vi "SaveSpec.vi"(3 "其它规格":T6={"其它勾选类规格"={"保存图片"=FALSE, "上传设备状态数据"=FALSE, "保存数据"=FALSE, "开机默认开启监控摄像头"=FALSE, "启用mark拍照 "=FALSE}, "其它数据类规格"={"相机1像素-毫米换算系数"=15.0, "相机2像素-毫米换算系数"=15.0, "D盘剩余空间预警(G)"=15.0, "视频最长录制时间(秒)"=15.0}, "相机名称"={"相机1名称"="cam1", "相机2名称"="cam1", "Cam1启用"=FALSE, "Cam2启用"=FALSE, "Basler1"=FALSE, "Basler2"=FALSE}, "参数"={"Mark1曝光时间"=500, "Mark2曝光时间"=500, "二维码曝光时间"=500}} {"其它数据类规格"."视频最长录制时间(秒)" format="%.3f"; "其它数据类规格"."D盘剩余空间预警(G)" format="%.3f"; "其它数据类规格"."相机1像素-毫米换算系数" format="%.5f"; "其它数据类规格"."相机2像素-毫米换算系数" format="%.5f"}) -> (0 "File out":path)   [LabVIEW 2014]
uses:
  Controls/OtherSpec.ctl
  <vilib>/userdefined/High Color/IMAQdx.ctl
  Global.vi
  <vilib>/Utility/file.llb/Write To Spreadsheet File (string).vi
panel:
  out "输出数组":string[][](array[string])
  in  "参数":T1={"Mark1曝光时间"=500.0, "Mark2曝光时间"=500.0, "二维码曝光时间"=500.0}
  in  "相机名称":T2={"相机1名称"="cam1", "相机2名称"="cam1", "Cam1启用"=FALSE, "Cam2启用"=FALSE, "Basler1"=FALSE, "Basler2"=FALSE}
  in  "其它数据类规格":T4={"相机1像素-毫米换算系数"=15.0, "相机2像素-毫米换算系数"=15.0, "D盘剩余空间预警(G)"=15.0, "视频最长录制时间(秒)"=15.0} {"视频最长录制时间(秒)" format="%.3f"; "D盘剩余空间预警(G)" format="%.3f"; "相机1像素-毫米换算系数" format="%.5f"; "相机2像素-毫米换算系数" format="%.5f"}
  in  "其它勾选类规格":T5
  out "输出字符串 3":string
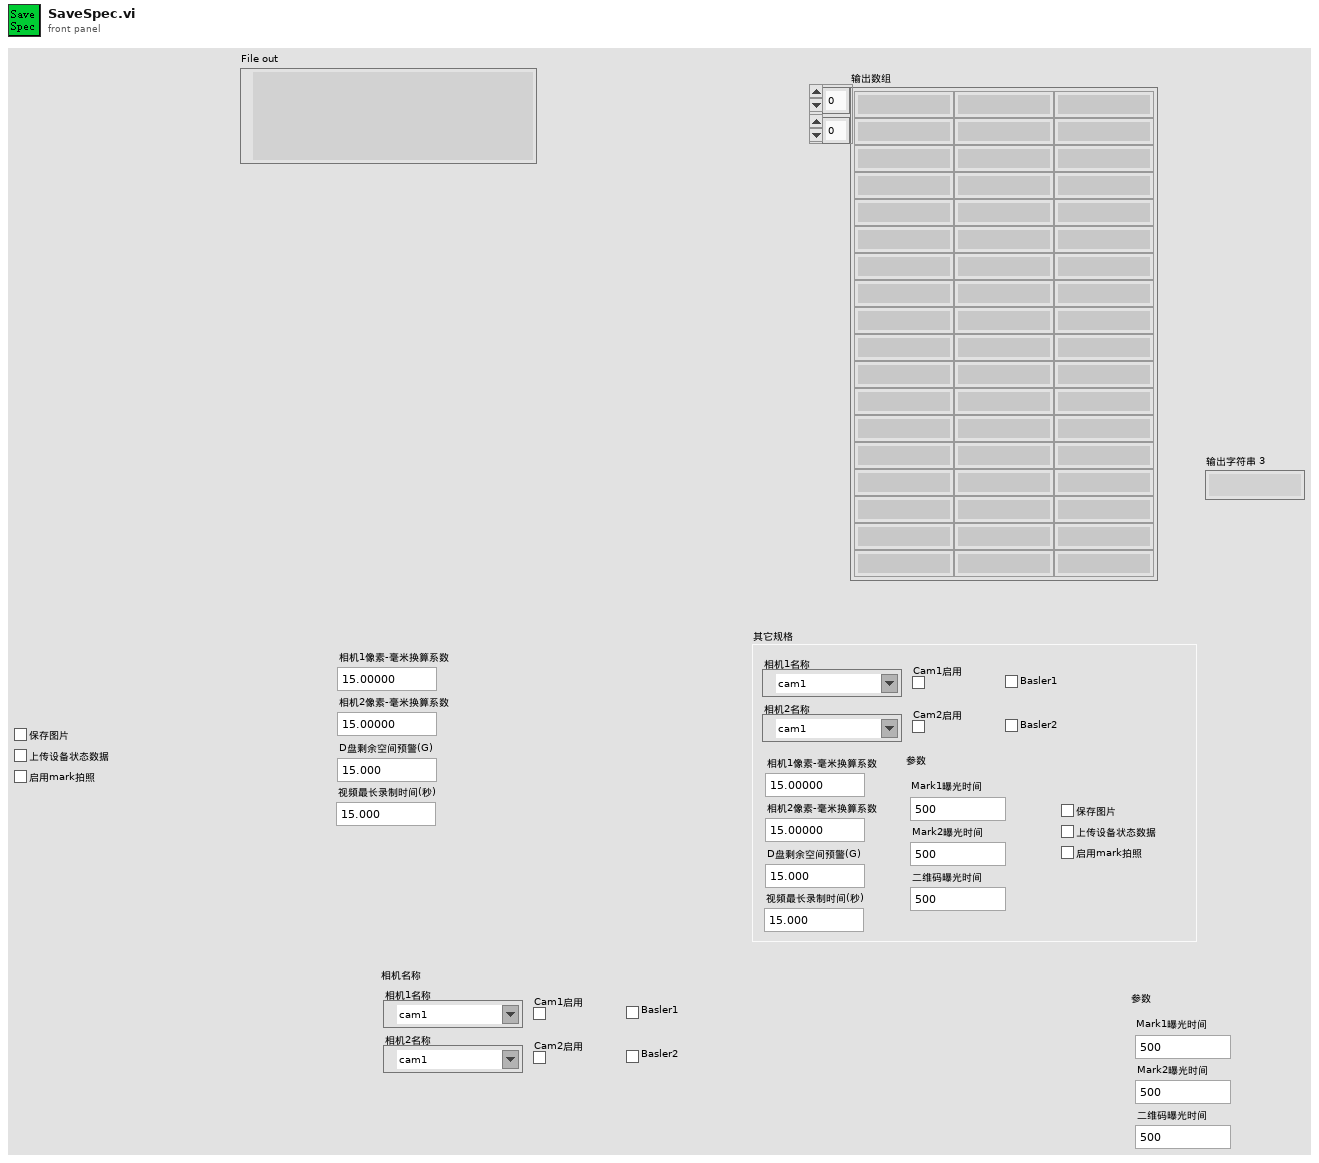
[diagram p1: front panel]
types:
  T1 = cluster{"Mark1曝光时间":dbl, "Mark2曝光时间":dbl, "二维码曝光时间":dbl}
  T2 = typedef "相机名称品牌使用状态.ctl" = cluster{"相机1名称":T3, "相机2名称":T3, "Cam1启用":bool, "Cam2启用":bool, "Basler1":bool, "Basler2":bool}
  T3 = typedef "IMAQdx.ctl" = refnum<k21>
  T4 = typedef "其他数据类规格.ctl" = cluster{"相机1像素-毫米换算系数":dbl, "相机2像素-毫米换算系数":dbl, "D盘剩余空间预警(G)":dbl, "视频最长录制时间(秒)":dbl}
  T5 = typedef "其它勾选类规格.ctl" = cluster{"保存图片":bool, "上传设备状态数据":bool, "保存数据":bool, "开机默认开启监控摄像头":bool, "启用mark拍照 ":bool}
  T6 = typedef "OtherSpec.ctl" = cluster{"其它勾选类规格":T5, "其它数据类规格":T4, "相机名称":T2, "参数":cluster{"Mark1曝光时间":i32, "Mark2曝光时间":i32, "二维码曝光时间":i32}}
  T7 = cluster{"Mark1曝光时间":i32, "Mark2曝光时间":i32, "二维码曝光时间":i32}
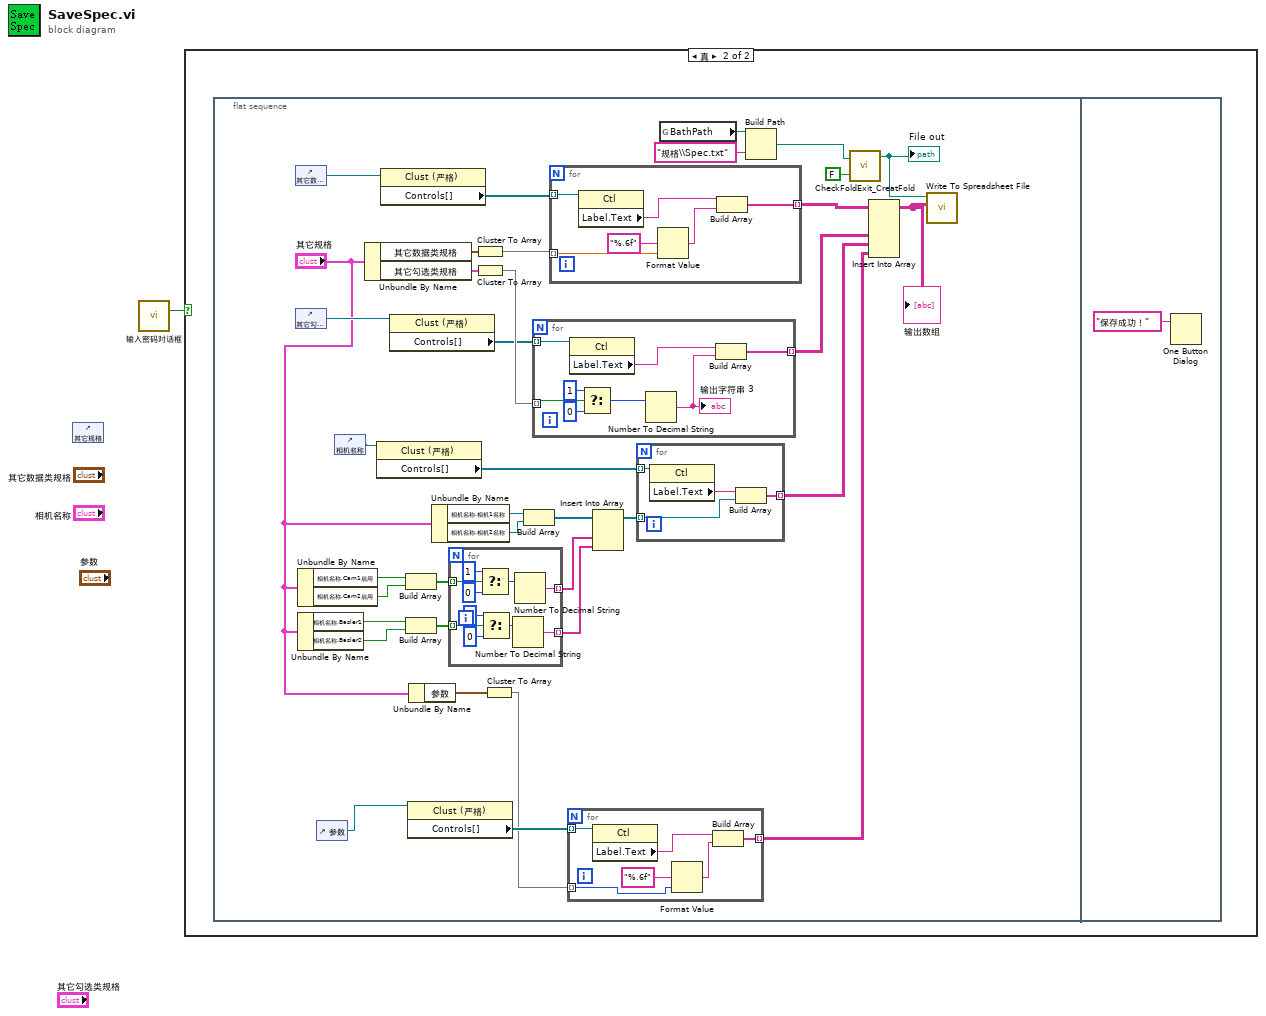
[diagram p0: block diagram]
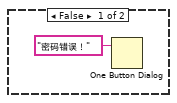
[diagram p2: hidden frame]
diagram:
  n1 = control-ref of="其它规格"() -> ()  [unwired: 1 out]
  n2 = call "输入密码对话框.vi"() -> ("密码正确"=w1:bool)  [unwired: 11 in]
  n3 = case shown="真" w1 {
    frame False {
      n4 = One Button Dialog(message="密码错误！" ("消息")) -> ()  [unwired: 1 in, 1 out]
    }
    frame True {
      n5 = flat-sequence {
        frame #0 {
          n6 = control-ref of="其它数据类规格"() -> (w26:refnum<vi>)
          n7 = control-ref of="其它勾选类规格"() -> (w29:refnum<vi>)
          n8 = Unbundle By Name("其它规格") -> ("相机名称.Cam1启用"=w19:bool, "相机名称.Cam2启用"=w20:bool)
          n9 = Unbundle By Name("其它规格") -> ("相机名称.Basler1"=w17:bool, "相机名称.Basler2"=w16:bool)
          n10 = control-ref of="参数"() -> (w5:refnum<vi>)
          n11 = control-ref of="相机名称"() -> (w23:refnum<vi>)
          n12 = Unbundle By Name("其它规格") -> ("其它数据类规格"=w32:T4, "其它勾选类规格"=w31:T5)
          n13 = property class="Clust (严格)"(reference=w23) -> ("Controls[]"=w18:refnum<vi>[])  [unwired: 1 in, 2 out]
          n14 = property class="Clust (严格)"(reference=w26) -> ("Controls[]"=w27:refnum<vi>[])  [unwired: 1 in, 2 out]
          n15 = property class="Clust (严格)"(reference=w29) -> ("Controls[]"=w28:refnum<vi>[])  [unwired: 1 in, 2 out]
          n16 = Build Array(w19, w20) -> (w14:bool[])
          n17 = Build Array(w17, w16) -> (w15:bool[])
          n18 = property class="Clust (严格)"(reference=w5) -> ("Controls[]"=w8:refnum<vi>[])  [unwired: 1 in, 2 out]
          n19 = Unbundle By Name("其它规格") -> ("参数"=w9:T7)
          n20 = Unbundle By Name("其它规格") -> ("相机名称.相机1名称"=w22:T3, "相机名称.相机2名称"=w21:T3)
          n21 = for {
            tunnel: [w52] -> w11 mode=indexing
            tunnel: w15 -> [w51] mode=indexing
            tunnel: w14 -> [w47] mode=indexing
            tunnel: [w46] -> w12 mode=indexing
            n22 = Select(t=1, s=w47, f=0 ("t")) -> (s? t:f=w50:i32)
            n23 = Select(t=1, s=w51, f=0 ("t")) -> (s? t:f=w53:i32)
            n24 = Number To Decimal String(number=w53) -> (decimal integer string=w52:string)  [unwired: 1 in]
            n25 = Number To Decimal String(number=w50) -> (decimal integer string=w46:string)  [unwired: 1 in]
          }
          n26 = Cluster To Array(cluster=w32) -> (array=w34:dbl[])
          n27 = Cluster To Array(cluster=w31) -> (array=w30:bool[])
          n28 = Cluster To Array(cluster=w9) -> (array=w4:i32[])
          n29 = Build Array(w22, w21) -> (w13:T3[])
          n30 = for {
            tunnel: [w66] -> w24 mode=indexing
            tunnel: w28 -> [w67] mode=indexing
            tunnel: w30 -> [w65] mode=indexing
            n31 = property class="Ctl"(reference=w67) -> ("Label.Text"=w60:string)  [unwired: 1 in, 2 out]
            n32 = Select(t=1, s=w65, f=0 ("t")) -> (s? t:f=w62:i32)
            n33 = Number To Decimal String(number=w62) -> (decimal integer string=w61:string)  [unwired: 1 in]
            "输出字符串 3" <- w61
            n34 = Build Array(w60, w61) -> (w66:string[])
          }
          n35 = for {
            tunnel: [w69] -> w25 mode=indexing
            tunnel: w27 -> [w73] mode=indexing
            tunnel: w34 -> [w71] mode=indexing
            n36 = property class="Ctl"(reference=w73) -> ("Label.Text"=w68:string)  [unwired: 1 in, 2 out]
            n37 = Format Value(format string="%.6f" ("format (%.3f)"), value (0)=w71) -> (output string=w70:string)  [unwired: 1 in]
            n38 = Build Array(w68, w70) -> (w69:string[])
          }
          n39 = for {
            tunnel: [w43] -> w3 mode=indexing
            tunnel: w8 -> [w45] mode=indexing
            tunnel: w4 -> [w40] mode=indexing
            n40 = property class="Ctl"(reference=w45) -> ("Label.Text"=w42:string)  [unwired: 1 in, 2 out]
            n41 = Format Value(format string="%.6f" ("format (%.3f)"), value (0)=w40) -> (output string=w44:string)  [unwired: 1 in]
            n42 = Build Array(w42, w44) -> (w43:string[])
          }
          n43 = Insert Into Array(array=w13, new element #1=w12, new element #2=w11) -> (w10:T3[])  [unwired: 1 in]
          n44 = for {
            tunnel: [w58] -> w6 mode=indexing
            tunnel: w18 -> [w59] mode=indexing
            tunnel: w10 -> [w56] mode=indexing
            n45 = property class="Ctl"(reference=w59) -> ("Label.Text"=w57:string)  [unwired: 1 in, 2 out]
            n46 = Build Array(w57, w56) -> (w58:string[])
          }
          n47 = global read "Global.vi" "BathPath"() -> (w37:path)
          n48 = Build Path(base path=w37, name or relative path="规格\\Spec.txt" ("名称或相对路径")) -> (appended path=w36:path)
          n49 = call "CheckFoldExit_CreatFold.vi"("path in"=w36, "FoldOrFile¡H"=FALSE) -> ("File out"=w38:path)  [unwired: 2 out]
          "File out" <- w38
          n50 = Insert Into Array(array=w25, new element #1=w24, new element #2=w6, new element #3=w3) -> (w33:string[][])  [unwired: 2 in]
          "输出数组" <- w33
          n51 = call-poly <vilib>:"Write To Spreadsheet File.vi"("2D data"=w33, "file path (dialog if empty)"=w38) -> ()  [unwired: 6 in, 1 out]
        }
        frame #1 {
          n52 = One Button Dialog(message="保存成功！" ("消息")) -> ()  [unwired: 1 in, 1 out]
        }
      }
    }
  }
